vi "GEA3 Write ERD (Rev 2 API) Multiple Messages.vi"(0 "GEA2 Reference In":refnum<k24>, 1 "# of Tries":u8=3 min=1 step=1, 2 "Read Timeout (ms)":u32=500, 5 "GEA Inputs":T1 {"Destination" format="%.0x"; "Source" format="%.0x"}, 7 "Write ERD List":T2[](array[typedef]) {"ERD Number" format="%.0x"}, 11 "Error In":errorcluster, 13 "Verify ERD Response?":bool=TRUE) -> (4 "GEA2 Reference Out":refnum<k24>, 8 "Raw Data Out":string[](array[string]), 15 "Error Out":errorcluster)   [LabVIEW 2018, in "GEA2_Toolkit.lvlib"]
uses:
  C:/Users/iallatyp/Desktop/New folder/GEA3/library/GEA2_Toolkit.lvlib
  type defs/ERD Write Data In.ctl
  type defs/Data Type.ctl
  D:/Common/LabVIEW GEA2 Toolkit/source/GEA3 DLL Source/GeaCommunication.dll
  source/GEA3 DLL Source/GeaCommunication.dll
  type defs/Source_Destination.ctl
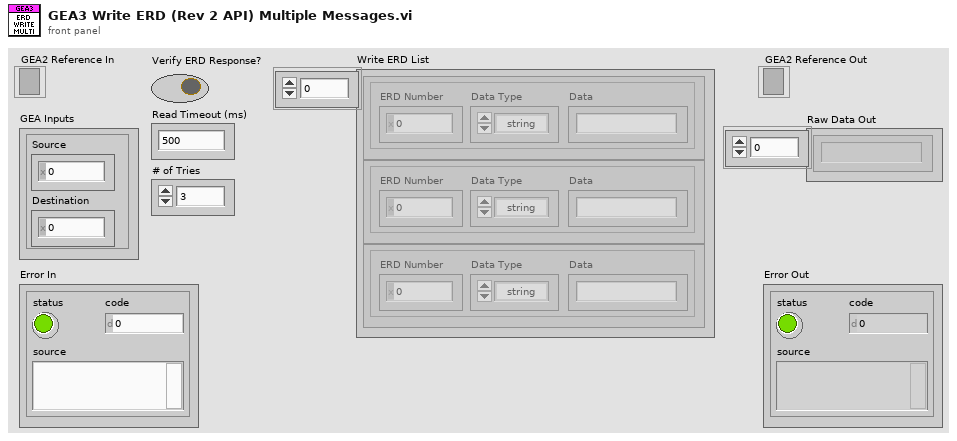
[diagram p1: front panel]
types:
  T1 = typedef "GEA2_Toolkit.lvlib/Source_Destination.ctl" = cluster{"Source":u8, "Destination":u8}
  T2 = typedef "GEA2_Toolkit.lvlib/ERD Write Data In.ctl" = cluster{"ERD Number":u16, "Data Type":T3, "Data":string}
  T3 = typedef "GEA2_Toolkit.lvlib/Data Type.ctl" = enum16{"string", "boolean", "uint8_t", "uint16_t", "uint32_t", "uint64_t", "int8_t", "int16_t", "int32_t", "int64_t"}
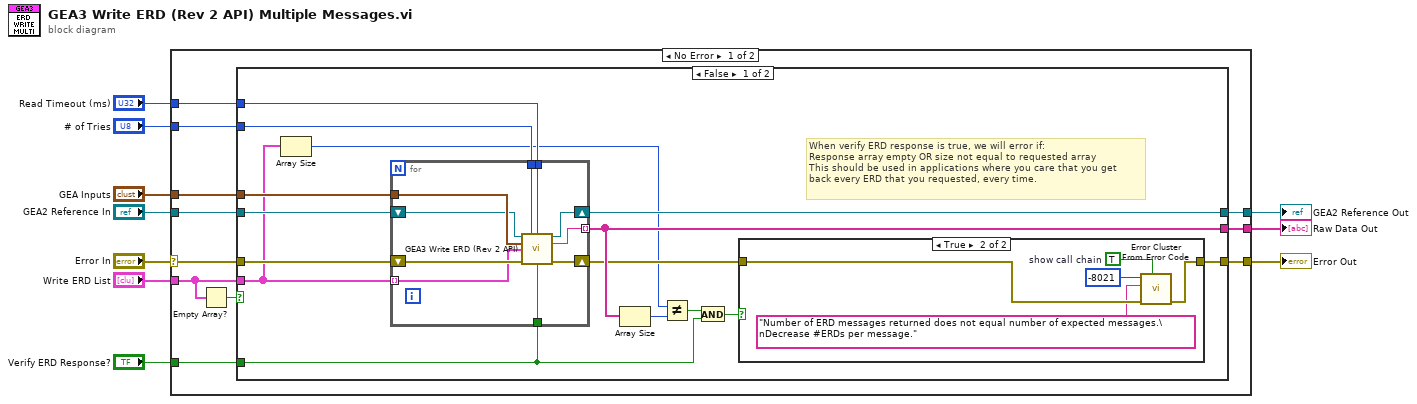
[diagram p0: block diagram]
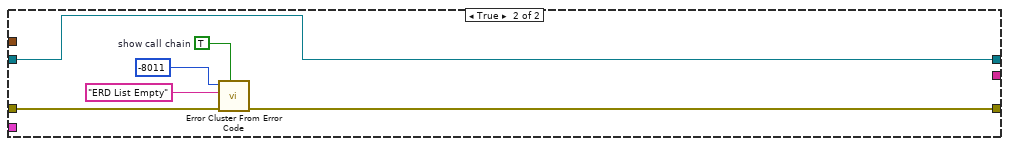
[diagram p3: hidden frame]
diagram:
  n1 = case shown="No Error" "Error In" {
    selector: "Error In" -> [w11 w60]
    tunnel: [w21 w59] -> w10
    tunnel: [w20 w60] -> w9
    tunnel: "Verify ERD Response?" -> [w19 _]
    tunnel: "GEA Inputs" -> [w18 _]
    tunnel: "Read Timeout (ms)" -> [w17 _]
    tunnel: "# of Tries" -> [w16 _]
    tunnel: "GEA2 Reference In" -> [w15 w59]
    tunnel: [w14 _] -> w3
    tunnel: "Write ERD List" -> [w12 _]
    frame No Error {
      n2 = Empty Array?(array=w12) -> (empty?=w13:bool)
      n3 = case shown="False" w13 {
        tunnel: [w26 w53] -> w21
        tunnel: w11 -> [w36 w55]
        tunnel: [w29 w54] -> w20
        tunnel: w19 -> [w25 _]
        tunnel: w18 -> [w35 _]
        tunnel: w17 -> [w34 _]
        tunnel: w16 -> [w33 _]
        tunnel: w15 -> [w32 w53]
        tunnel: w12 -> [w31 _]
        tunnel: [w28 _] -> w14
        frame False {
          # "When verify ERD response is true, we will error if:\nResponse array empty OR size not equal to requested array\nThis should be used in applications where you care that you get\nback every ERD that you requested, every time."
          n4 = Array Size(array=w31) -> (size(s)=w22:i32)
          n5 = for {
            tunnel: w25 -> [w49]
            tunnel: w35 -> [w48]
            tunnel: [w47] -> w28 mode=indexing
            tunnel: w34 -> [w46]
            tunnel: w33 -> [w44]
            shift-right: [w52] -> w26
            shift-left: w32 -> [w45]
            shift-right: [w50] -> w27
            shift-left: w36 -> [w51]
            tunnel: w31 -> [w43] mode=indexing
            n6 = call "GEA3 Write ERD (Rev 2 API).vi"("GEA2 Reference In"=w45, "# of Tries"=w44, "Read Timeout (ms)"=w46, "GEA Inputs"=w48, "ERD Write Data In"=w43, "Error In"=w51, "Verify ERD Response?"=w49) -> ("GEA2 Reference Out"=w52:refnum<k24>, "Raw Data Out"=w47:string, "Error Out"=w50:errorcluster)  [unwired: 6 in]
          }
          n7 = Array Size(array=w28) -> (size(s)=w30:i32)
          n8 = Not Equal?(x=w22, y=w30) -> (x != y?=w23:bool)
          n9 = And(x=w23, y=w25) -> (x .and. y?=w24:bool)
          n10 = case shown="True" w24 {
            tunnel: w27 -> [w37 w40]
            tunnel: [w37 w39] -> w29
            frame False {
            }
            frame True {
              w42 = TRUE  # show call chain
              n11 = call <vilib>:"Error Cluster From Error Code.vi"("show call chain? (False)"=w42, "error in (no error)"=w40, "error message (\"\")"="Number of ERD messages returned does not equal number of expected messages.\nDecrease #ERDs per message." ("error message (\"\")"), "error code (0)"=-8021) -> ("error out"=w39:errorcluster)  [unwired: 5 in]
            }
          }
        }
        frame True {
          w56 = TRUE  # show call chain
          n12 = call <vilib>:"Error Cluster From Error Code.vi"("show call chain? (False)"=w56, "error in (no error)"=w55, "error message (\"\")"="ERD List Empty" ("error message (\"\")"), "error code (0)"=-8011) -> ("error out"=w54:errorcluster)  [unwired: 5 in]
        }
      }
    }
    frame Error {
    }
  }
  "GEA2 Reference Out" <- w10
  "Error Out" <- w9
  "Raw Data Out" <- w3
